vi "GetAccessors.vi"(8 "error in (no error)":errorcluster, 9 "AccessorType":T1, 11 "ClassReflector in":refnum<class "ClassReflector.lvclass">) -> (0 "error out":errorcluster, 2 "AccessorInfo":T2[](array[typedef]), 3 "ClassReflector out":refnum<class "ClassReflector.lvclass">)   [LabVIEW 2023, in "ClassReflector.lvclass"]
uses:
  ClassReflector.lvclass
  AccessorInfoCluster.ctl
  AccessorTypeEnum.ctl
  ClassReflector.lvclass/ClassReflector.ctl
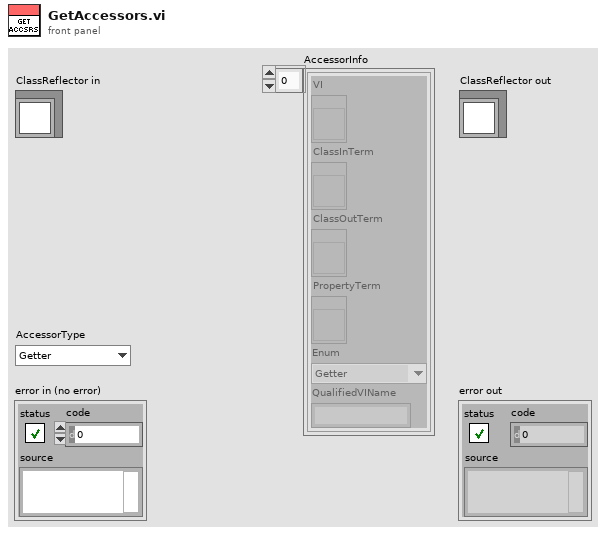
[diagram p1: front panel]
types:
  T1 = typedef "ClassReflector.lvclass/AccessorTypeEnum.ctl" = enum16{"Getter", "Setter"}
  T2 = typedef "ClassReflector.lvclass/AccessorInfoCluster.ctl" = cluster{"VI":refnum<vi>, "ClassInTerm":refnum<vi>, "ClassOutTerm":refnum<vi>, "PropertyTerm":refnum<vi>, "Enum":T1, "QualifiedVIName":string}
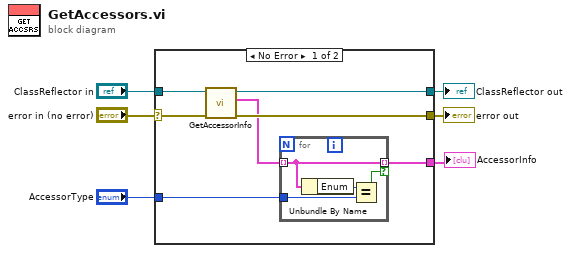
[diagram p0: block diagram]
diagram:
  n1 = case shown="No Error" "error in (no error)" {
    selector: "error in (no error)" -> [w10 w19]
    tunnel: [w12 w19] -> w5
    tunnel: [w13 w18] -> w3
    tunnel: "ClassReflector in" -> [w11 w18]
    tunnel: [w8 _] -> w2
    tunnel: "AccessorType" -> [w7 _]
    frame No Error {
      n2 = call "GetAccessorInfo.vi"("error in (no error)"=w10, "ClassReflector in"=w11) -> ("error out"=w12:errorcluster, "AccessorInfo"=w9:T2[], "ClassReflector out"=w13:refnum<class "ClassReflector.lvclass">)  [unwired: 7 in]
      n3 = for {
        tunnel: w9 -> [w16] mode=indexing
        tunnel: [w16] -> w8 mode=indexing if=w15
        tunnel: w7 -> [w14]
        n4 = Unbundle By Name(w16) -> ("Enum"=w17:T1)
        n5 = Equal?(x=w17, y=w14) -> (x = y?=w15:bool)
      }
    }
    frame Error {
    }
  }
  "error out" <- w5
  "ClassReflector out" <- w3
  "AccessorInfo" <- w2
